vi "SaveFromMemory.vi"(8 "error in (no error)":errorcluster, 10 "Data_2_Save":T1(array[cluster]), 11 "DBAL-BIN in":refnum<class "DBAL-BIN.lvclass">) -> (0 "error out":errorcluster, 3 "DBAL-BIN out":refnum<class "DBAL-BIN.lvclass">)   [LabVIEW 2020, in "Sgraph_lib_V1.lvlib" / "DBAL-BIN.lvclass"]
doc: "Must override!"
uses:
  DBAL-BIN.lvclass
  DBAL-BIN.lvclass/DBAL-BIN.ctl
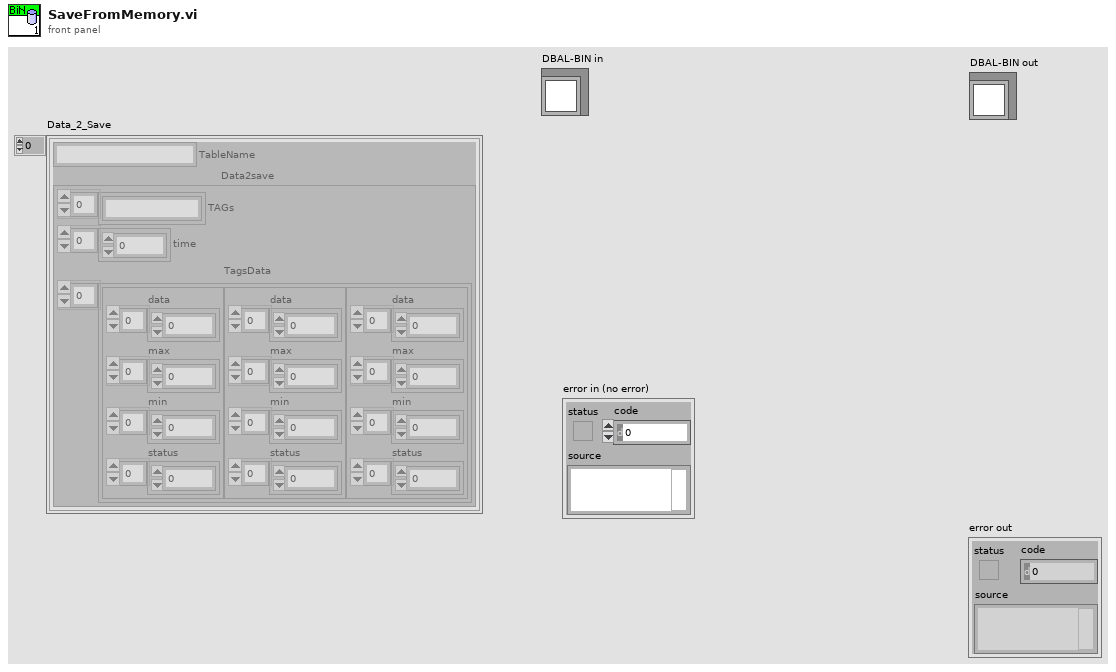
[diagram p1: front panel]
types:
  T1 = cluster{"TableName":string, "Data2save":cluster{"TAGs":string[], "time":dbl[], "TagsData":cluster{"data":dbl[], "max":dbl[], "min":dbl[], "status":u32[]}[]}}[]
  T2 = typedef "Sgraph_lib_V1.lvlib/DBAL-BIN.lvclass/BinFolderPace.ctl" = enum16{"PerDay", "PerWeek", "PerYear"}
  T3 = typedef "Sgraph_lib_V1.lvlib/DBAL.lvclass/DBAL_PAQ_TimeRange.ctl" = cluster{"Tmax":dbl, "Tmin":dbl}
  T4 = cluster{"TableName":string, "Data2save":cluster{"TAGs":string[], "time":dbl[], "TagsData":cluster{"data":dbl[], "max":dbl[], "min":dbl[], "status":u32[]}[]}}
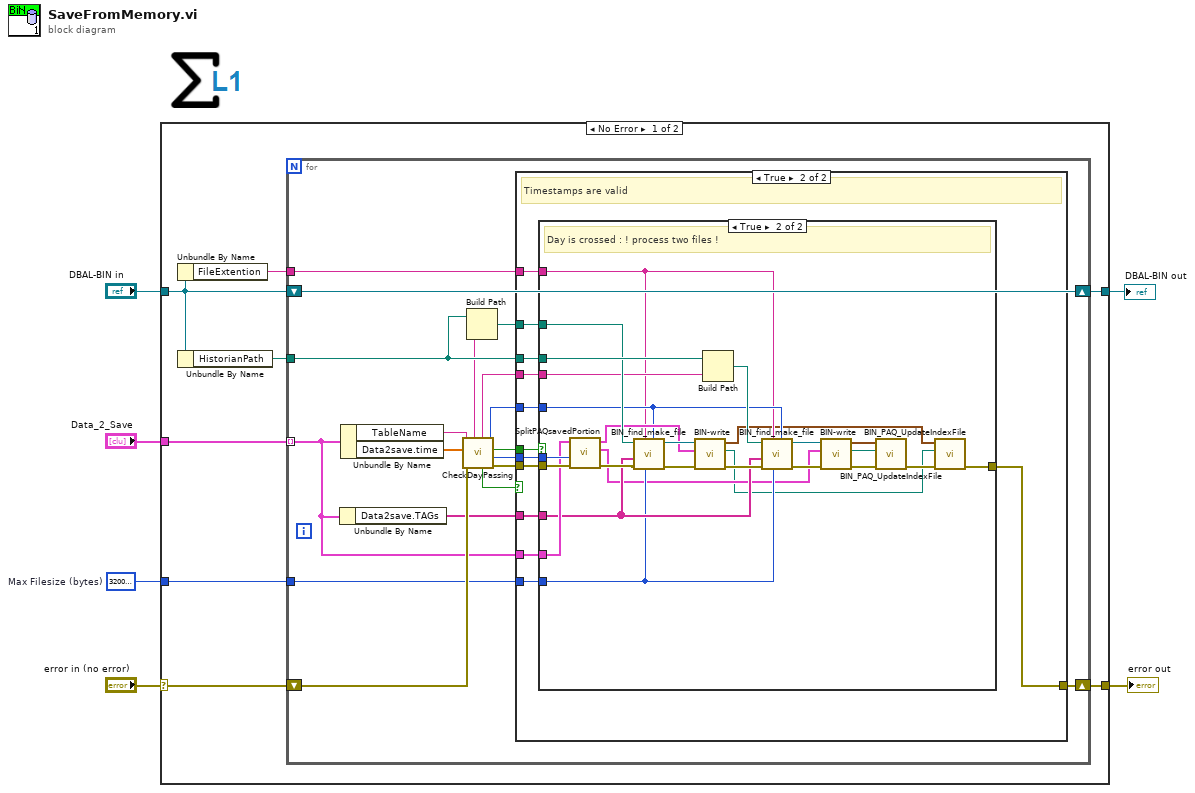
[diagram p0: block diagram]
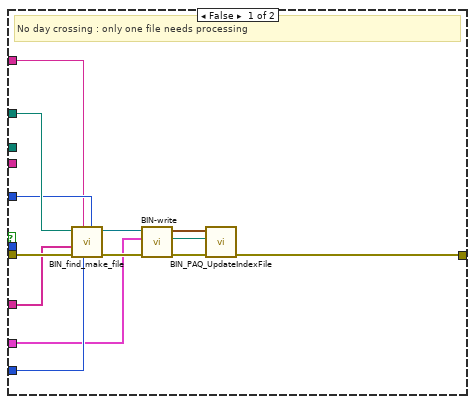
[diagram p3: hidden frame]
diagram:
  w1 = i64 32000000  # Max Filesize (bytes)
  n1 = case shown="No Error" "error in (no error)" {
    selector: "error in (no error)" -> [w14 w86]
    tunnel: [w12 w86] -> w5
    tunnel: "DBAL-BIN in" -> [w9 w85]
    tunnel: [w13 w85] -> w3
    tunnel: "Data_2_Save" -> [w11 _]
    tunnel: w1 -> [w7 _]
    frame No Error {
      n2 = Unbundle By Name(w9) -> ("FileExtention"=w8:string)
      n3 = Unbundle By Name(w9) -> ("HistorianPath"=w10:path)
      n4 = for {
        shift-right: [w15] -> w13
        shift-left: w9 -> [w15]
        shift-right: [w16] -> w12
        shift-left: w14 -> [w28]
        tunnel: w11 -> [w20] mode=indexing
        tunnel: w10 -> [w23]
        tunnel: w8 -> [w25]
        tunnel: w7 -> [w24]
        n5 = Unbundle By Name(w20) -> ("Data2save.TAGs"=w19:string[])
        n6 = Unbundle By Name(w20) -> ("TableName"=w22:string, "Data2save.time"=w31:dbl[])
        n7 = call "CheckDayPassing.vi"("error in"=w28, "Data2save.time"=w31, "TableName"=w22) -> ("error out"=w32:errorcluster, "split-index"=w29:i32, "Split array"=w30:bool, "FolderPace"=w18:T2, "TimeValid"=w21:bool, "PeriodName2"=w27:string, "PeriodName1"=w17:string)  [unwired: 2 in]
        n8 = Build Path(base path=w23, name or relative path=w17) -> (appended path=w26:path)
        n9 = case shown="True" w21 {
          tunnel: w32 -> [w33 w45]
          tunnel: w20 -> [_ w44]
          tunnel: w30 -> [_ w35]
          tunnel: w29 -> [_ w43]
          tunnel: w27 -> [_ w42]
          tunnel: w26 -> [_ w41]
          tunnel: w25 -> [_ w40]
          tunnel: w24 -> [_ w39]
          tunnel: w23 -> [_ w38]
          tunnel: w19 -> [_ w37]
          tunnel: w18 -> [_ w36]
          tunnel: [w33 w34] -> w16
          frame False {
            # "Invalid timestamp !"
          }
          frame True {
            # "Timestamps are valid"
            n10 = case shown="True" w35 {
              tunnel: w44 -> [w52 w82]
              tunnel: w45 -> [w58 w83]
              tunnel: w43 -> [_ w84]
              tunnel: [w49 w65] -> w34
              tunnel: w38 -> [_ w81]
              tunnel: w42 -> [_ w63]
              tunnel: w41 -> [w57 w74]
              tunnel: w40 -> [w47 w62]
              tunnel: w39 -> [w56 w71]
              tunnel: w37 -> [w55 w72]
              tunnel: w36 -> [w51 w68]
              frame False {
                # "No day crossing : only one file needs processing"
                n11 = call "BIN_find_make_file.vi"("FolderPace"=w51, "Max Filesize (bytes)"=w56, "Extension"=w47, "error in"=w58, "TAGs"=w55, "OpenPattern"=w57) -> ("error out"=w54:errorcluster, "refnum out"=w53:refnum<file>)  [unwired: 3 in, 1 out]
                n12 = call "BIN-write.vi"("error in"=w54, "Data in"=w52, "refnum in"=w53) -> ("error out"=w50:errorcluster, "path"=w46:path, "TimeRange"=w48:T3)  [unwired: 6 in]
                n13 = call "BIN_PAQ_UpdateIndexFile.vi"("error in (no error)"=w50, "path"=w46, "TimeRange"=w48) -> ("error out"=w49:errorcluster)  [unwired: 8 in]
              }
              frame True {
                # "Day is crossed : ! process two files !"
                n14 = call "SplitPAQsavedPortion.vi"("error in"=w83, "split-index"=w84, "SaveData in"=w82) -> ("error out"=w79:errorcluster, "SaveData out Day2"=w69:T4, "SaveData out Day1"=w70:T4)  [unwired: 6 in]
                n15 = call "BIN_find_make_file.vi"("FolderPace"=w68, "Max Filesize (bytes)"=w71, "Extension"=w62, "error in"=w79, "TAGs"=w72, "OpenPattern"=w74) -> ("error out"=w78:errorcluster, "refnum out"=w80:refnum<file>)  [unwired: 3 in, 1 out]
                n16 = call "BIN-write.vi"("error in"=w78, "Data in"=w70, "refnum in"=w80) -> ("error out"=w75:errorcluster, "path"=w59:path, "TimeRange"=w61:T3)  [unwired: 6 in]
                n17 = Build Path(base path=w81, name or relative path=w63) -> (appended path=w73:path)
                n18 = call "BIN_find_make_file.vi"("FolderPace"=w68, "Max Filesize (bytes)"=w71, "Extension"=w62, "error in"=w75, "TAGs"=w72, "OpenPattern"=w73) -> ("error out"=w77:errorcluster, "refnum out"=w76:refnum<file>)  [unwired: 3 in, 1 out]
                n19 = call "BIN-write.vi"("error in"=w77, "Data in"=w69, "refnum in"=w76) -> ("error out"=w67:errorcluster, "path"=w60:path, "TimeRange"=w64:T3)  [unwired: 6 in]
                n20 = call "BIN_PAQ_UpdateIndexFile.vi"("error in (no error)"=w67, "path"=w60, "TimeRange"=w64) -> ("error out"=w66:errorcluster)  [unwired: 8 in]
                n21 = call "BIN_PAQ_UpdateIndexFile.vi"("error in (no error)"=w66, "path"=w59, "TimeRange"=w61) -> ("error out"=w65:errorcluster)  [unwired: 8 in]
              }
            }
          }
        }
      }
    }
    frame Error {
    }
  }
  "error out" <- w5
  "DBAL-BIN out" <- w3
